vi "FourFlippingCoins13.vi"() -> ()   [LabVIEW 2013]
panel:
  in  "Number of Trials":dbl
  out "Number of Heads":dbl
  out "Coin 4":bool
  out "Coin 3":bool
  out "Coin 2":bool
  out "Coin 1":bool
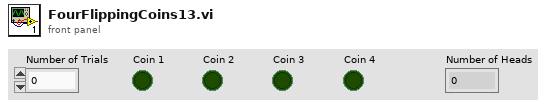
[diagram p1: front panel]
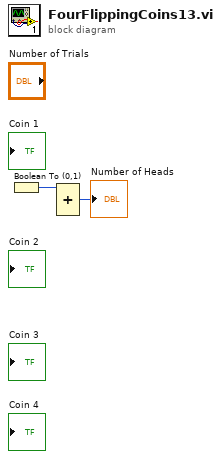
[diagram p0: block diagram]
diagram:
  n1 = Boolean To (0,1)() -> (0, 1=w1:i16)  [unwired: 1 in]
  n2 = Compound Arithmetic op=ADD(w1) -> (→"Number of Heads":i16)  [unwired: 3 in]
